vi "am2305_3.vi"() -> ()   [LabVIEW 2024]
uses:
  <vilib>/Utility/NIReport.llb/Report Type.ctl
  <vilib>/Instr/_visa.llb/VISA Configure Serial Port (Instr).vi
  <vilib>/addons/_office/excel.llb/Excel Easy Table (str).vi
  <vilib>/Utility/NIReport.llb/NI_report.lvclass
  <vilib>/Utility/NIReport.llb/NI_ReportGenerationCore.lvlib
  <vilib>/addons/_office/NI_ReportGenerationToolkit.lvlib
  <vilib>/Utility/NIReport.llb/Excel/NI_Excel.lvclass
panel:
  in  "Iniviar":bool
  out "RH  vs Date":waveform(dbl)(graph)
  out "Temperature vs Date":waveform(dbl)(graph)
  in  "VISA resource name":refnum<visa-resource-name>="COM8"
  in  "template (empty)":path
  out "Humedad Relativa actual\n(%)":dbl format="%#_6f"
  out "Temperatura actual\n(°C)":dbl format="%#_6f"
  in  "Parar":bool
  # "Adquisición de Datos: Humedad Relativa y Temperatura"
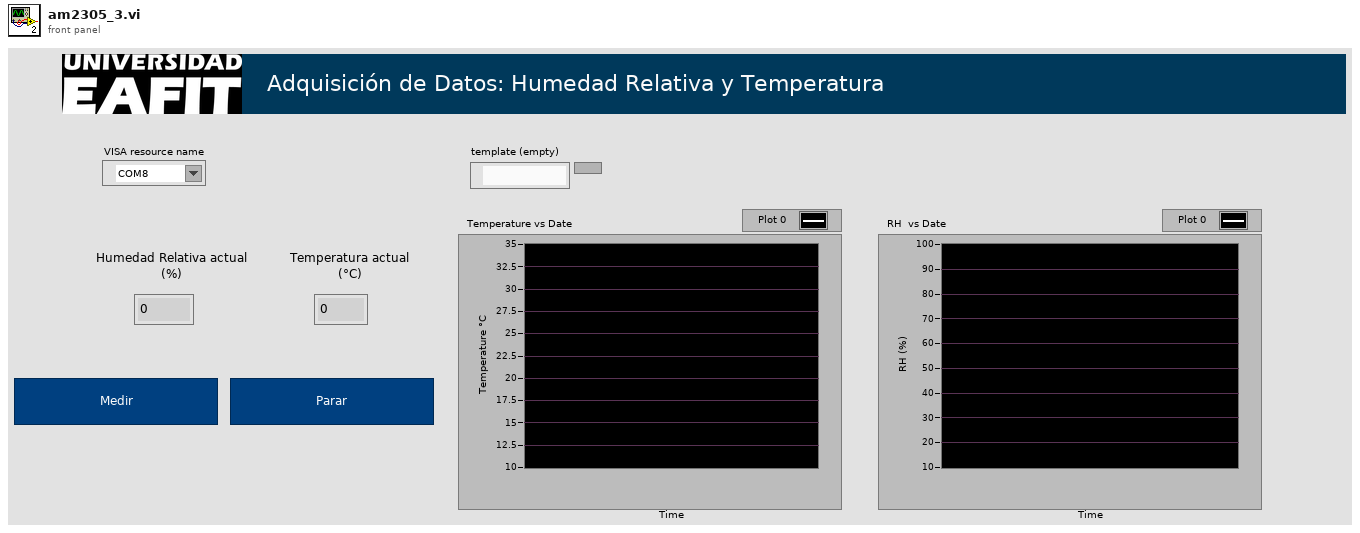
[diagram p1: front panel]
types:
  T1 = typedef "NI_ReportGenerationCore.lvlib/Report Type.ctl" = enum16{"HTML", "Word", "Excel"}
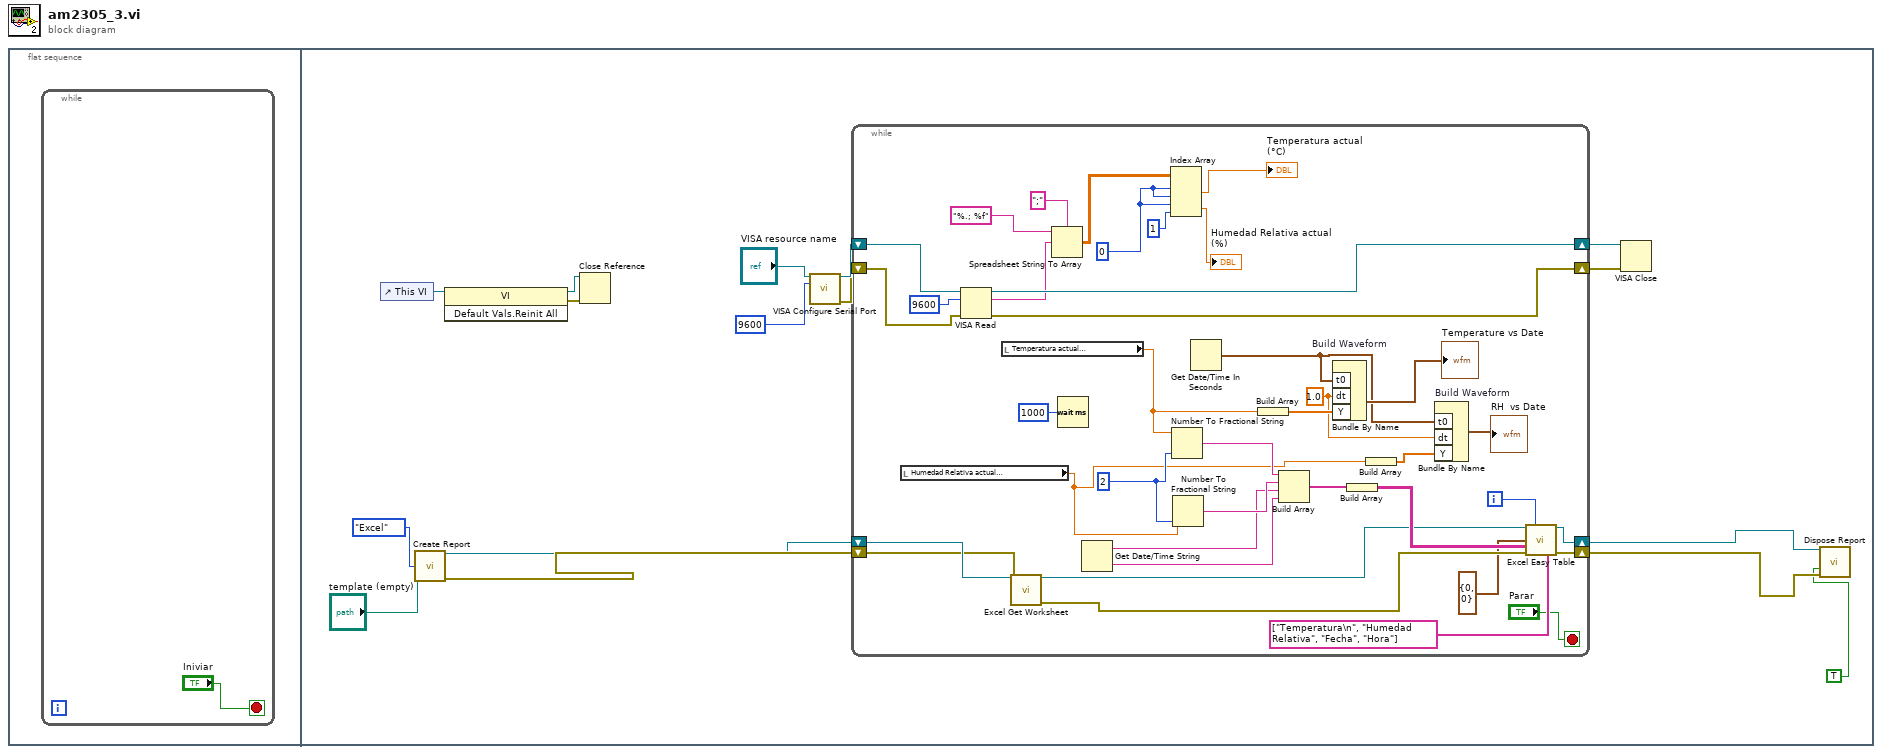
[diagram p0: block diagram]
diagram:
  n1 = flat-sequence {
    frame #0 {
      n2 = while {
        stop <- "Iniviar" stop-if-true
      }
    }
    frame #1 {
      n3 = control-ref of="This VI"() -> (w8:refnum<vi>)
      n4 = call <vilib>:"Create Report.vi"("report type"=Report_Type."Excel", "template (empty)"="template (empty)") -> ("report out"=w14:refnum<class "NI_report.lvclass">, "error out"=w15:errorcluster)  [unwired: 12 in]
      n5 = invoke class="VI" method="Default Vals.Reinit All"(reference=w8) -> (reference out=w9:refnum<vi>, error out=w10:errorcluster)  [unwired: 2 in, 1 out]
      n6 = Close Reference(reference=w9, error in (no error)=w10) -> ()  [unwired: 1 out]
      n7 = call-poly "VISA Configure Serial Port"("VISA resource name"="VISA resource name", "baud rate (9600)"=u32 9600) -> ("VISA resource name out"=w6:refnum<visa-resource-name>, "error out"=w2:errorcluster)  [unwired: 12 in]
      n8 = while {
        shift-right: [w48] -> w4
        shift-left: w6 -> [w49]
        shift-right: [w47] -> w3
        shift-left: w2 -> [w46]
        shift-right: [w45] -> w16
        shift-left: w14 -> [w43]
        shift-right: [w44] -> w17
        shift-left: w15 -> [w42]
        i -> [w26]
        stop <- "Parar" stop-if-true
        w21 = 0 ("index (row)")
        w32 = 1.0 ("dt")
        w50 = i16 2 ("precision (6)")
        n9 = local read "Humedad Relativa actual\n(%)"() -> (w31:dbl)
        n10 = VISA Read(VISA resource name=w49, byte count=u32 9600, error in (no error)=w46) -> (VISA resource name out=w48:refnum<visa-resource-name>, read buffer=w25:string, error out=w47:errorcluster)  [unwired: 1 out]
        n11 = local read "Temperatura actual\n(°C)"() -> (w37:dbl)
        n12 = call <vilib>:"Excel Get Worksheet.vi"("report in"=w43, "error in (no error)"=w42) -> ("report out"=w40:refnum<class "NI_report.lvclass">, "error out"=w41:errorcluster)  [unwired: 12 in]
        n13 = Spreadsheet String To Array(delimiter (Tab)=";", format string="%.; %f", spreadsheet string=w25) -> (array=w22:dbl[][])  [unwired: 1 in]
        n14 = Wait (ms)(milliseconds to wait=u32 1000) -> ()  [unwired: 1 out]
        n15 = Get Date/Time String() -> (date string=w39:string, time string=w38:string)  [unwired: 3 in]
        n16 = Index Array(array=w22, index (row) #1=w21, index (col) #1=w21, index (row) #2=w21, index (col) #2=1 ("disabled index (col)")) -> (element #1=→"Temperatura actual\n(°C)":dbl, element #2=→"Humedad Relativa actual\n(%)":dbl)
        n17 = Number To Fractional String(number=w37, precision (6)=w50) -> (F-format string=w52:string)  [unwired: 2 in]
        n18 = Number To Fractional String(number=w31, precision (6)=w50) -> (F-format string=w53:string)  [unwired: 2 in]
        n19 = Get Date/Time In Seconds() -> (seconds since 1Jan1904=w33:timestamp)
        n20 = Build Array(w37) -> (w36:dbl[])
        n21 = Build Array(w52, w53, w39, w38) -> (w54:string[])
        n22 = Bundle By Name "Build Waveform"("t0"=w33, "dt"=w32, "Y"=w36) -> (→"Temperature vs Date":waveform(dbl))  [unwired: 1 in]
        n23 = Build Array(w54) -> (w55:string[][])
        n24 = Build Array(w31) -> (w30:dbl[])
        n25 = Bundle By Name "Build Waveform"("t0"=w33, "dt"=w32, "Y"=w30) -> (→"RH  vs Date":waveform(dbl))  [unwired: 1 in]
        n26 = call-poly <vilib>:"Excel Easy Table.vi"("report in"=w40, "iteration"=w26, "start (0, 0)"=cluster{"row":i32, "column":i32} {"row"=0, "column"=0}, "text data"=w55, "error in (no error)"=w41, "column headers"=string[] ["Temperatura\n", "Humedad Relativa", "Fecha", "Hora"]) -> ("report out"=w45:refnum<class "NI_report.lvclass">, "error out"=w44:errorcluster)  [unwired: 5 in, 3 out]
      }
      n27 = VISA Close(VISA resource name=w4, error in (no error)=w3) -> ()  [unwired: 1 out]
      n28 = call-dynamic "Dispose Report.vi"("report in"=w16, "save changes? (F)"=TRUE, "error in (no error)"=w17) -> ()  [unwired: 12 in, 1 out]
    }
  }
